vi "Write battery status file.vi"(7 "Application path":path, 8 "Error In":errorcluster, 10 "Battery voltage":dbl, 11 "MAC address":string) -> (0 "Error Out":errorcluster, 3 "Result":string)   [LabVIEW 2016]
uses:
  <vilib>/Utility/file.llb/Read Delimited Spreadsheet (string).vi
  <vilib>/Utility/file.llb/Write Delimited Spreadsheet (string).vi
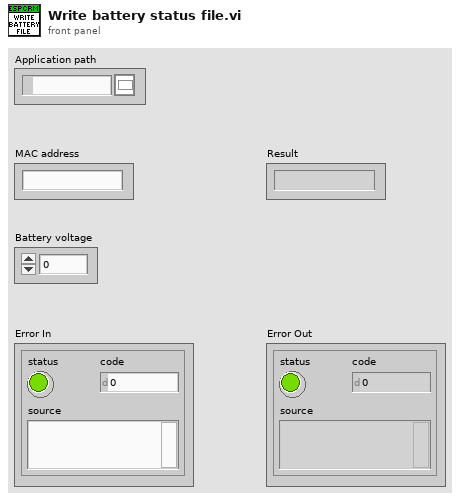
[diagram p1: front panel]
types:
  T1 = enum16{"open", "replace", "create", "open or create", "replace or create", "replace or create with confirmation"}
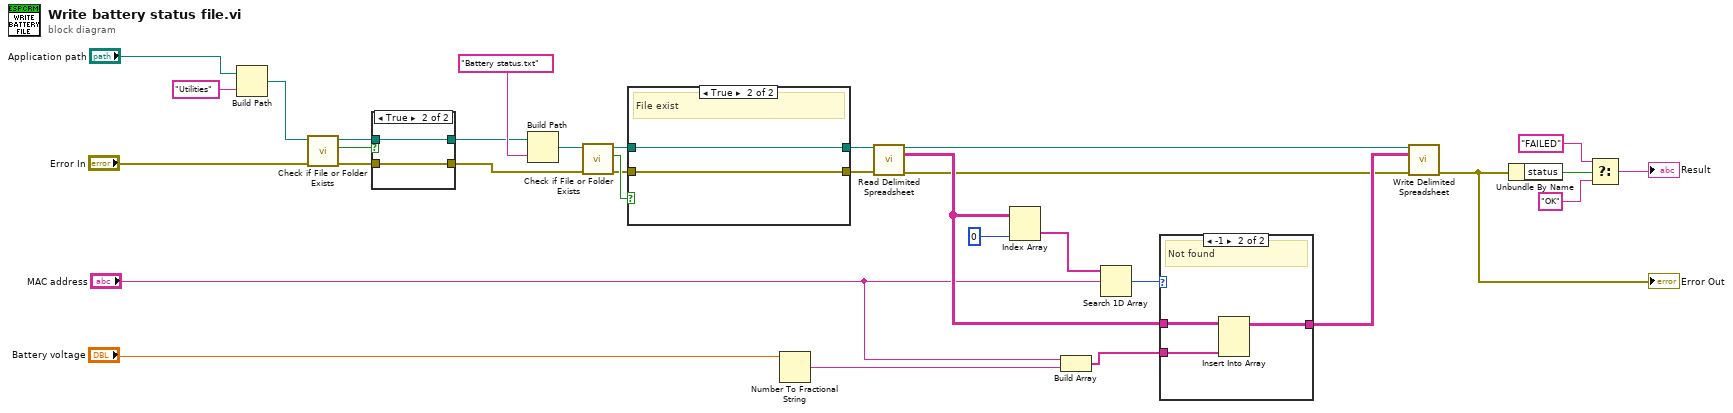
[diagram p0: block diagram]
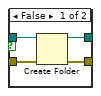
[diagram p2: hidden frame]
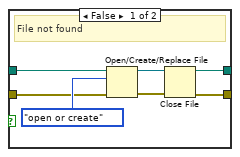
[diagram p3: hidden frame]
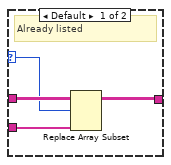
[diagram p4: hidden frame]
diagram:
  n1 = Build Path(base path="Application path", name or relative path="Utilities") -> (appended path=w17:path)
  n2 = call <vilib>:"Check if File or Folder Exists.vi"("error in (no error)"="Error In", "path"=w17) -> ("error out"=w16:errorcluster, "file or folder exists?"=w14:bool, "dup path"=w15:path)  [unwired: 7 in]
  n3 = case shown="True" w14 {
    tunnel: w16 -> [w36 w37]
    tunnel: w15 -> [w35 w38]
    tunnel: [w34 w38] -> w12
    tunnel: [w33 w37] -> w11
    frame False {
      n4 = Create Folder(path (use dialog)=w35, error in=w36) -> (created path=w34:path, error out=w33:errorcluster)  [unwired: 1 in, 1 out]
    }
    frame True {
    }
  }
  n5 = Build Path(base path=w12, name or relative path="Battery status.txt" ("string")) -> (appended path=w21:path)
  n6 = call <vilib>:"Check if File or Folder Exists.vi"("error in (no error)"=w11, "path"=w21) -> ("error out"=w18:errorcluster, "file or folder exists?"=w20:bool, "dup path"=w19:path)  [unwired: 7 in]
  n7 = case shown="True" w20 {
    tunnel: [w42 w47] -> w23
    tunnel: [w41 w46] -> w22
    tunnel: w19 -> [w40 w47]
    tunnel: w18 -> [w39 w46]
    frame False {
      # "File not found"
      n8 = Open/Create/Replace File(file path (use dialog)=w40, error in=w39, operation (0:open)=T1."open or create") -> (refnum out=w43:refnum<file>, error out=w44:errorcluster)  [unwired: 3 in, 1 out]
      n9 = Close File(refnum=w43, error in=w44) -> (path=w42:path, error out=w41:errorcluster)
    }
    frame True {
      # "File exist"
    }
  }
  n10 = Number To Fractional String(number="Battery voltage") -> (F-format string=w27:string)  [unwired: 3 in]
  n11 = call-poly <vilib>:"Read Delimited Spreadsheet.vi"("file path (dialog if empty)"=w23, "error in (no error)"=w22) -> ("new file path (Not A Path if cancelled)"=w25:path, "all rows"=w28:string[][], "error out"=w7:errorcluster)  [unwired: 8 in, 3 out]
  n12 = Index Array(array=w28, index (col)=0 ("disabled index (col)")) -> (element=w30:string[])  [unwired: 1 in]
  n13 = Build Array("MAC address", w27) -> (w26:string[])
  n14 = Search 1D Array(1D array=w30, element="MAC address") -> (index of element=w29:i32)  [unwired: 1 in]
  n15 = case shown="-1" w29 {
    selector: w29 -> [w49 _]
    tunnel: w28 -> [w51 w54]
    tunnel: w26 -> [w50 w53]
    tunnel: [w48 w52] -> w24
    frame Default {
      # "Already listed"
      n16 = Replace Array Subset(array=w51, new element=w50, index (row)=w49) -> (w48:string[][])  [unwired: 1 in]
    }
    frame -1 {
      # "Not found"
      n17 = Insert Into Array(array=w54, new element=w53) -> (w52:string[][])  [unwired: 2 in]
    }
  }
  n18 = call-poly <vilib>:"Write Delimited Spreadsheet.vi"("file path (dialog if empty)"=w25, "2D data"=w24, "error in (no error)"=w7) -> ("error out"=w3:errorcluster)  [unwired: 11 in, 1 out]
  "Error Out" <- w3
  n19 = Unbundle By Name(w3) -> ("status"=w6:bool)
  n20 = Select(t="FAILED", s=w6, f="OK") -> (s? t:f=→"Result":string)
